vi "data claster to array.vi"(11 "Cluster":T1) -> (3 "Array":u64[](array[numeric]))   [LabVIEW 2021]
uses:
  pdw.ctl
  mode_type.ctl
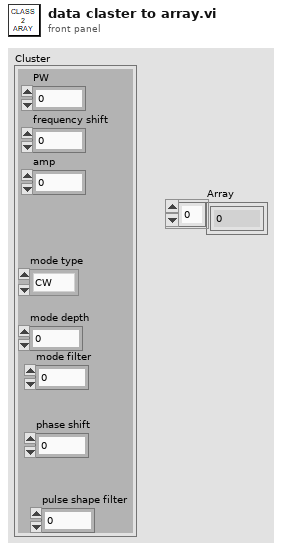
[diagram p1: front panel]
types:
  T1 = typedef "pdw.ctl" = cluster{"PW":u32, "frequency shift":fxp<+/-,48,0>, "amp":fxp<+/-,18,1>, "mode type":T2, "mode depth":u32, "mode filter":u8, "phase shift":fxp<+/-,16,1>, "pulse shape filter":u8}
  T2 = typedef "mode_type.ctl" = enum8{"CW", "NC - CW", "NC - cw", "LFM", "BPSK", "QPSK"}
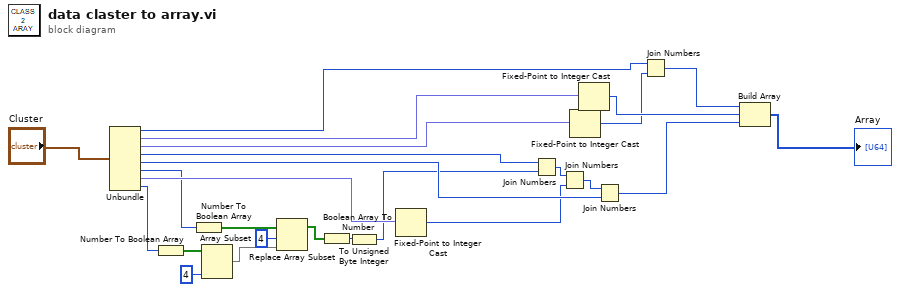
[diagram p0: block diagram]
diagram:
  n1 = Unbundle("Cluster") -> ("PW"=w20:u32, "frequency shift"=w18:fxp<+/-,48,0>, "amp"=w19:fxp<+/-,18,1>, "mode type"=w17:T2, "mode depth"=w13:u32, "mode filter"=w10:u8, "phase shift"=w12:fxp<+/-,16,1>, "pulse shape filter"=w9:u8)
  n2 = Number To Boolean Array(number=w9) -> (Boolean array=w8:bool[])
  n3 = Number To Boolean Array(number=w10) -> (Boolean array=w6:bool[])
  n4 = Array Subset(array=w8, length=4) -> (w5:bool[])  [unwired: 1 in]
  n5 = Replace Array Subset(array=w6, new element=w5, index=4) -> (w3:bool[])
  n6 = Boolean Array To Number(Boolean array=w3) -> (number=w2:u32)
  n7 = To Unsigned Byte Integer(number=w2) -> (unsigned 8bit integer=w1:u8)
  n8 = Fixed-Point to Integer Cast(1:w12) -> (0:w11:i16)
  n9 = Join Numbers(hi=w17, lo=w1) -> ((hi.lo)=w16:u16)
  n10 = Join Numbers(hi=w16, lo=w11) -> ((hi.lo)=w15:u32)
  n11 = Fixed-Point to Integer Cast(1:w19) -> (0:w21:i32)
  n12 = Fixed-Point to Integer Cast(1:w18) -> (0:w23:i64)
  n13 = Join Numbers(hi=w15, lo=w13) -> ((hi.lo)=w14:u64)
  n14 = Join Numbers(hi=w20, lo=w21) -> ((hi.lo)=w22:u64)
  n15 = Build Array(w22, w23, w14) -> (→"Array":u64[])
